vi "AcquireEventDigitizerV1729A.vi"(8 "error in (no error)":errorcluster, 10 "handle in":i32, 11 "VME Base Address":u32) -> (0 "error out":errorcluster, 3 "handle out":i32)   [LabVIEW 2014]
uses:
  Program Files (x86)/CAEN/Comm/labview/CAENComm.lvlib
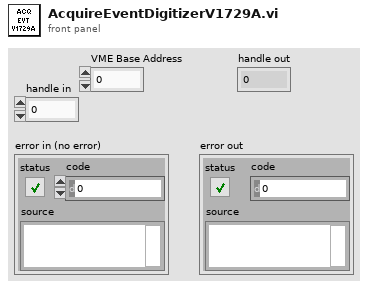
[diagram p1: front panel]
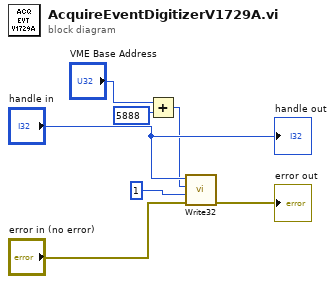
[diagram p0: block diagram]
diagram:
  n1 = Add(x="VME Base Address", y=u32 5888 ("x")) -> (x+y=w4:u32)
  n2 = call "Write32.vi"("error in (no error)"="error in (no error)", "Data"=u32 1, "Address"=w4, "handle"="handle in") -> ("error out"=→"error out":errorcluster)  [unwired: 7 in]
  "handle out" <- "handle in"
